vi "SourceChangeEvent.vi"(4 "SourceChangeEvent":refnum<user-event>, 5 "Event Data":cluster{"sender":refnum<k24>, "e":refnum<k24>}, 6 "Control Ref":refnum<k24>, 7 "Event Common Data":T1) -> ()   [LabVIEW 2020, in "LcWebView.lvclass"]
uses:
  LcWebView.lvclass
  C:/Projects/WebView2/LcWebView/data/Microsoft.Web.WebView2.Core.dll
  data/Microsoft.Web.WebView2.Core.dll
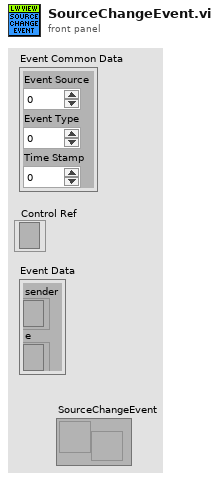
[diagram p1: front panel]
types:
  T1 = cluster{"Event Source":i32, "Event Type":u32, "Time Stamp":u32}
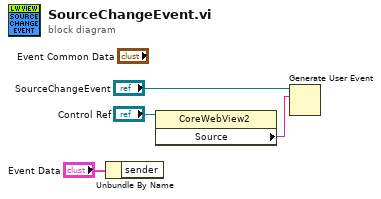
[diagram p0: block diagram]
diagram:
  n1 = Unbundle By Name("Event Data") -> ()  [unwired: 1 out]
  n2 = property class="CoreWebView2"(reference="Control Ref") -> ("Source"=w1:string)  [unwired: 1 in, 2 out]
  n3 = Generate User Event(user event="SourceChangeEvent", event data cluster=w1) -> ()  [unwired: 2 in, 2 out]
